vi "D.vi"(1 "Ts":dbl, 2 "e[k-1]":dbl, 3 "e[k]":dbl) -> (0 "d":dbl)   [LabVIEW 2011]
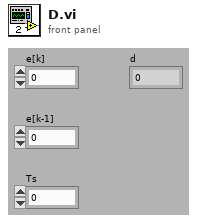
[diagram p1: front panel]
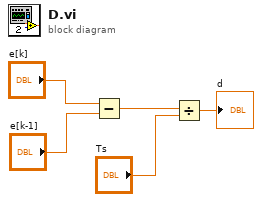
[diagram p0: block diagram]
diagram:
  n1 = Subtract(x="e[k]", y="e[k-1]") -> (x-y=w3:dbl)
  n2 = Divide(x=w3, y="Ts") -> (x/y=→"d":dbl)
